vi "PLC.vi"(11 "Idx":i32) -> ()   [LabVIEW 2016]
doc: "Sound Analyzer queued state machine"
uses:
  PLC.Data.ctl
  PLC.Data.Status.ctl
  PLC.State.ctl
  PLC.Data.Sets.ctl
  LowLevel/PLC.DataBlock.PCstatus.ctl
  LowLevel/PLC.DataBlock.PCstatus.General.ctl
  LowLevel/PLC.DataBlock.PCstatus.Station.ctl
  LowLevel/PLC.DataBlock.PLCstatus.ctl
  LowLevel/PLC.DataBlock.PLCstatus.General.ctl
  LowLevel/PLC.DataBlock.PLCstatus.Station.ctl
  PLC.Action.ctl
  tools/CitTemplate/citTemplate.errData.ctl
  tools/EventLog/EventLog.EventSource.ctl
  Database/Database.Global.vi
  PLC.Global.vi
panel:
  out "action":T1=enum."-- PLC --"
  out "error.action":string
  out "error":errorcluster
  out "Data":T2={"Status"={"Idx"=0, "ConnRef"=0, "State"=enum."Off", "LiveBitTimer"=timestamp(0 s since 1904-01-01)}, "Sets"={"Enable"=FALSE, "IP"="", "Rack"=0, "Slot"=10000, "LifeBitTimer_s"=0.0, "DataBlockAddr_PCStatus"=0, "DataBlockAddr_PLCStatus"=1, "DataBlockAddr_PLCNewData"=[], "DataBlockSize_PLCNewData"=[], "DataBlockAddr_PLCChangeOver"=[], "DataBlockSize_PLCChangeOver"=[], "DataBlockAddr_PCChangeOver"=[], "DataBlockAddr_PLCCheckStatus"=[], "DataBlockSize_PLCCheckStatus"=[], "DataBlockAddr_PCCheckStatus"=[], "System"=""}, "PCstatus"={"General"={"LifeBit"=FALSE, "DbRun"=FALSE}, "Stations"=[]}, "PLCstatus"={"General"={"LifeBit"=FALSE}, "Stations"=[]}}
  out "_loop":i32(ring)=4
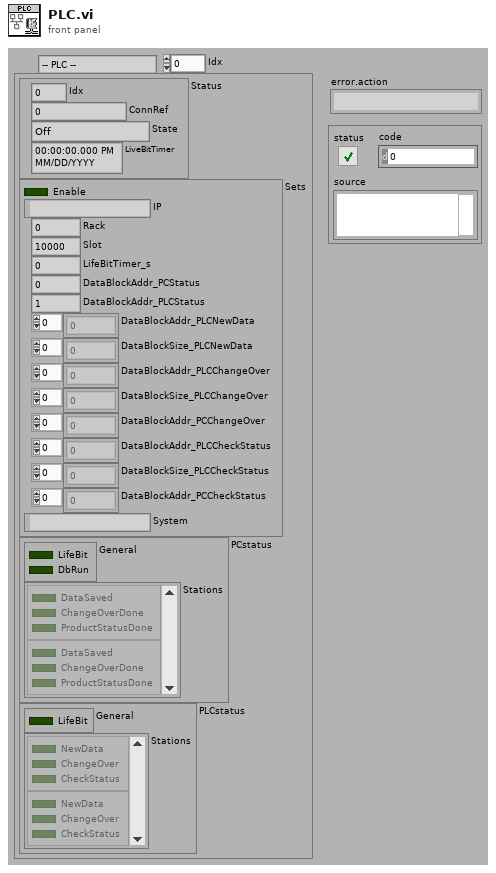
[diagram p1: front panel]
types:
  T1 = typedef "PLC.Action.ctl" = enum32{"idle", "constructor", "destructor", "-- PLC --", "Setup", "NewData", "ChangeOver", "CheckStatus"}
  T2 = typedef "PLC.Data.ctl" = cluster{"Status":T3, "Sets":T5, "PCstatus":T6, "PLCstatus":T9}
  T3 = typedef "PLC.Data.Status.ctl" = cluster{"Idx":i32, "ConnRef":u64, "State":T4, "LiveBitTimer":timestamp}
  T4 = typedef "PLC.State.ctl" = enum32{"Off", "Error", "Idle", "Run"}
  T5 = typedef "PLC.Data.Sets.ctl" = cluster{"Enable":bool, "IP":string, "Rack":i32, "Slot":i32, "LifeBitTimer_s":dbl, "DataBlockAddr_PCStatus":i32, "DataBlockAddr_PLCStatus":i32, "DataBlockAddr_PLCNewData":i32[], "DataBlockSize_PLCNewData":i32[], "DataBlockAddr_PLCChangeOver":i32[], "DataBlockSize_PLCChangeOver":i32[], "DataBlockAddr_PCChangeOver":i32[], "DataBlockAddr_PLCCheckStatus":i32[], "DataBlockSize_PLCCheckStatus":i32[], "DataBlockAddr_PCCheckStatus":i32[], "System":string}
  T6 = typedef "PLC.DataBlock.PCstatus.ctl" = cluster{"General":T7, "Stations":T8[]}
  T7 = typedef "PLC.DataBlock.PCstatus.General.ctl" = cluster{"LifeBit":bool, "DbRun":bool}
  T8 = typedef "PLC.DataBlock.PCstatus.Station.ctl" = cluster{"DataSaved":bool, "ChangeOverDone":bool, "ProductStatusDone":bool}
  T9 = typedef "PLC.DataBlock.PLCstatus.ctl" = cluster{"General":T10, "Stations":T11[]}
  T10 = typedef "PLC.DataBlock.PLCstatus.General.ctl" = cluster{"LifeBit":bool}
  T11 = typedef "PLC.DataBlock.PLCstatus.Station.ctl" = cluster{"NewData":bool, "ChangeOver":bool, "CheckStatus":bool}
  T12 = typedef "EventLog.EventSource.ctl" = enum16{"All", "Gui", "Ref", "File", "Arch", "Seq", "CPX", "DB", "Laser", "Scan.P", "Scan.O", "PLC"}
  T13 = typedef "citTemplate.errData.ctl" = cluster{"ts":timestamp, "src":T12, "instance":i32, "action":string, "error":errorcluster, "unconfirmed":bool}
  T14 = typedef "citTemplate.notifierHandle.ctl" = refnum<notifier>
  T15 = typedef "Database.Main.Data.Status.ctl" = cluster{"Run":bool, "Handle":i32, "ConnTS":timestamp, "DbTime":timestamp, "DbTimeCode":dbl, "DbTimeOffset":dbl}
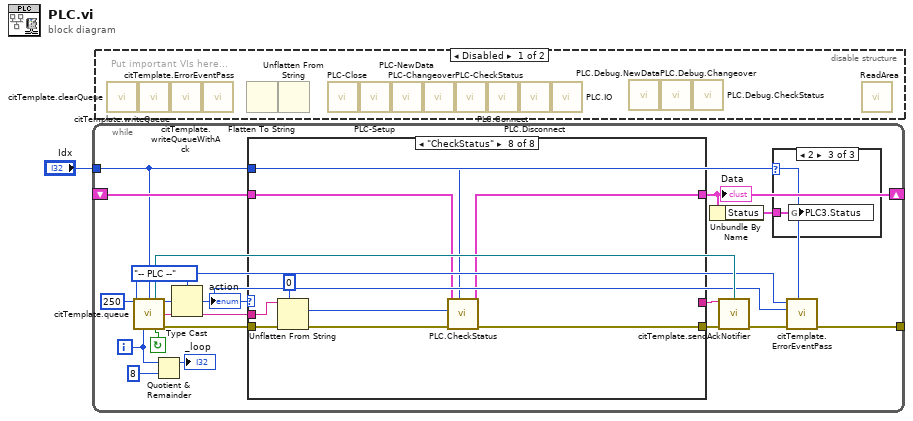
[diagram p0: block diagram]
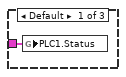
[diagram p2: hidden frame]
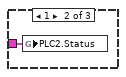
[diagram p3: hidden frame]
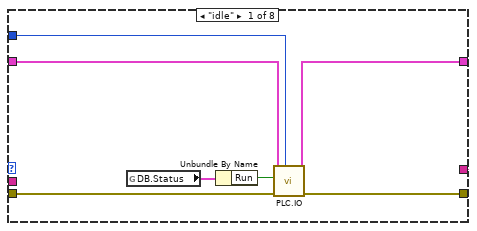
[diagram p4: hidden frame]
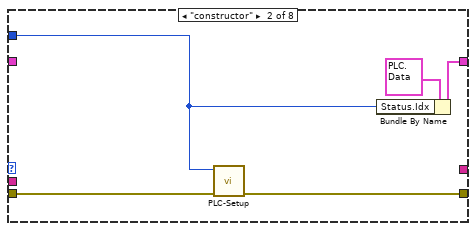
[diagram p5: hidden frame]
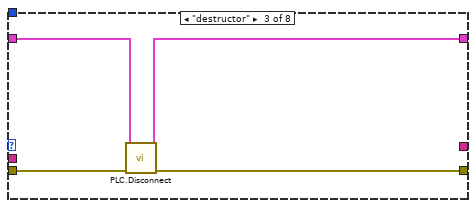
[diagram p6: hidden frame]
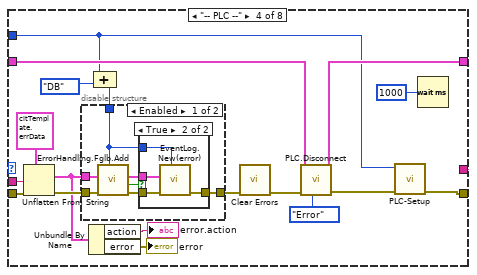
[diagram p7: hidden frame]
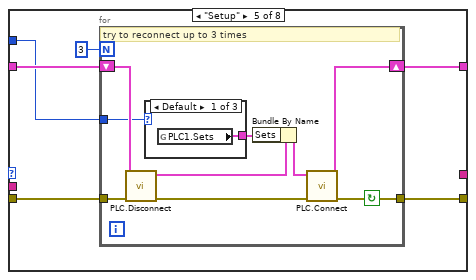
[diagram p10: hidden frame]
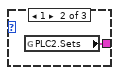
[diagram p11: hidden frame]
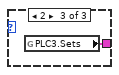
[diagram p12: hidden frame]
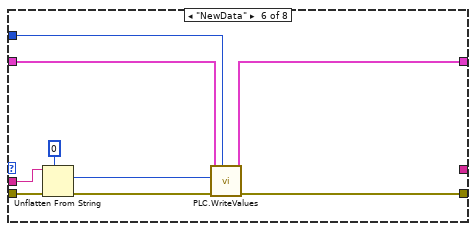
[diagram p13: hidden frame]
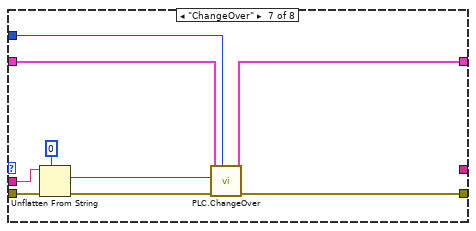
[diagram p14: hidden frame]
diagram:
  n1 = while {
    tunnel: [w9] -> _
    shift-right: [w6] -> _
    shift-left: _ -> [w7]
    tunnel: "Idx" -> [w2]
    i -> [w11]
    stop <- w16 continue-if-true
    w5 = PLC.Action."-- PLC --" ("Action")
    n2 = call "citTemplate.queue.vi"("ms timeout (250 ms)"=250, "instance (0)"=w2, "event enum"=w5, "iteration (-1)"=w11) -> ("notifierHandle out"=w15:T14, "event out"=w19:u32, "(flatten) data out"=w18:string, "continue"=w16:bool, "error out"=w17:errorcluster)  [unwired: 1 in, 6 out]
    n3 = Quotient & Remainder(x=w11, y=8) -> (x-y*floor(x/y)=→"_loop":i32)  [unwired: 1 out]
    n4 = Type Cast(type=w5, x=w19) -> (*(type *) &x=w10:T1)
    "action" <- w10
    n5 = case shown="\"CheckStatus\"" w10 {
      tunnel: w18 -> [_ _ _ w50 _ w91 w99 w108]
      tunnel: w17 -> [w28 w35 w39 w51 w76 w97 w101 w110]
      tunnel: ["" _ _ "" _ _ _ _] -> w14
      tunnel: [w27 w34 w38 w46 w75 w96 w106 w115] -> w4
      tunnel: [w26 w32 w36 w47 w74 w94 w104 w113] -> w6
      tunnel: w7 -> [w29 _ w37 w48 w73 w95 w105 w114]
      tunnel: w2 -> [w25 w31 _ w42 w71 w93 w103 w112]
      frame "idle" {
        n6 = global read "Database.Global.vi" "DB.Status"() -> (w24:T15)
        n7 = Unbundle By Name(w24) -> ("Run"=w23:bool)
        n8 = call "PLC.IO.vi"("Idx"=w25, "error in"=w28, "DbRun"=w23, "Data_in"=w29) -> ("error out"=w27:errorcluster, "Data_out"=w26:T2)  [unwired: 6 in]
      }
      frame "constructor" {
        n9 = call "PLC-Setup.vi"("error in"=w35, "Idx"=w31) -> ("error out"=w34:errorcluster)  [unwired: 9 in]
        n10 = Bundle By Name(cluster=T2 {"Status"={"Idx"=0, "ConnRef"=0, "State"=enum."Off", "LiveBitTimer"=timestamp(0 s since 1904-01-01)}, "Sets"={"Enable"=FALSE, "IP"="", "Rack"=0, "Slot"=10000, "LifeBitTimer_s"=0.0, "DataBlockAddr_PCStatus"=0, "DataBlockAddr_PLCStatus"=0, "DataBlockAddr_PLCNewData"=[], "DataBlockSize_PLCNewData"=[], "DataBlockAddr_PLCChangeOver"=[], "DataBlockSize_PLCChangeOver"=[], "DataBlockAddr_PCChangeOver"=[], "DataBlockAddr_PLCCheckStatus"=[], "DataBlockSize_PLCCheckStatus"=[], "DataBlockAddr_PCCheckStatus"=[], "System"=""}, "PCstatus"={"General"={"LifeBit"=FALSE, "DbRun"=FALSE}, "Stations"=[]}, "PLCstatus"={"General"={"LifeBit"=FALSE}, "Stations"=[]}} ("Data"), "Status.Idx"=w31) -> (w32:T2)
      }
      frame "destructor" {
        n11 = call "PLC.Disconnect.vi"("error in (no error)"=w39, "Data"=w37) -> ("error out"=w38:errorcluster, "Data out"=w36:T2)  [unwired: 8 in]
      }
      frame "-- PLC --" {
        n12 = Unflatten From String(type=T13 {"ts"=timestamp(0 s since 1904-01-01), "src"=enum."All", "instance"=0, "action"="", "error"={"status"=FALSE, "code"=0, "source"=""}, "unconfirmed"=FALSE} ("ErrData"), binary string=w50, error in (no error)=w51) -> (value=w54:T13, error out=w55:errorcluster)  [unwired: 2 in, 1 out]
        n13 = Unbundle By Name(w54) -> ("action"=→"error.action":string, "error"=→"error":errorcluster)
        n14 = Compound Arithmetic op=ADD(w42, EventLog.EventSource."DB" ("Event source")) -> (w41:i32)
        n15 = disable-structure shown="Enabled" {
          disable-tunnel: w55 -> [w64 w70]
          disable-tunnel: w54 -> [w63 _]
          disable-tunnel: [w62 w70] -> w49
          disable-tunnel: w41 -> [w59 _]
          frame Enabled {
            n16 = call "ErrorHandling.Fglb.Add.vi"("Event source"=w59, "error in (no error)"=w64, "Error in"=w63) -> ("error out"=w61:errorcluster, "changed?"=w60:bool)  [unwired: 7 in]
            n17 = case shown="True" w60 {
              tunnel: [w65 w69] -> w62
              tunnel: w63 -> [_ w68]
              tunnel: w61 -> [w65 w67]
              tunnel: w59 -> [_ w66]
              frame False {
              }
              frame True {
                n18 = call "EventLog.New(error).vi"("Source (All)"=w66, "error in"=w67, "ErrData"=w68) -> ("error out"=w69:errorcluster)  [unwired: 8 in]
              }
            }
          }
          frame Disabled {
          }
        }
        n19 = call <vilib>:"Clear Errors.vi"("error in (no error)"=w49) -> ("error out"=w43:errorcluster)  [unwired: 5 in, 1 out]
        n20 = call "PLC.Disconnect.vi"("State (Off)"=PLC.State."Error", "error in (no error)"=w43, "Data"=w48) -> ("error out"=w45:errorcluster, "Data out"=w47:T2)  [unwired: 7 in]
        n21 = call "PLC-Setup.vi"("error in"=w45, "Idx"=w42) -> ("error out"=w46:errorcluster)  [unwired: 9 in]
        n22 = Wait (ms)(milliseconds to wait=u32 1000) -> ()  [unwired: 1 out]
      }
      frame "Setup" {
        n23 = for {
          N: 3 -> [_]
          tunnel: w76 -> [w85]
          tunnel: [w78] -> w75
          shift-right: [w83] -> w74
          shift-left: w73 -> [w82]
          tunnel: w71 -> [w77]
          stop <- w78 continue-if-true
          # "try to reconnect up to 3 times"
          n24 = call "PLC.Disconnect.vi"("error in (no error)"=w85, "Data"=w82) -> ("error out"=w84:errorcluster, "Data out"=w80:T2)  [unwired: 8 in]
          n25 = case shown="Default" w77 {
            tunnel: [w86 w87 w88] -> w81
            frame Default {
              n26 = global read "PLC.Global.vi" "PLC1.Sets"() -> (w86:T5)
            }
            frame 1 {
              n27 = global read "PLC.Global.vi" "PLC2.Sets"() -> (w87:T5)
            }
            frame 2 {
              n28 = global read "PLC.Global.vi" "PLC3.Sets"() -> (w88:T5)
            }
          }
          n29 = Bundle By Name(cluster=w80, "Sets"=w81) -> (w79:T2)
          n30 = call "PLC.Connect.vi"("error in (no error)"=w84, "Data"=w79) -> ("error out"=w78:errorcluster, "Data out"=w83:T2)  [unwired: 8 in]
        }
      }
      frame "NewData" {
        n31 = Unflatten From String(type=0 ("Slot"), binary string=w91, error in (no error)=w97) -> (value=w89:i32, error out=w92:errorcluster)  [unwired: 2 in, 1 out]
        n32 = call "PLC.WriteValues.vi"("Idx"=w93, "error in"=w92, "Slot"=w89, "Data_in"=w95) -> ("error out"=w96:errorcluster, "Data_out"=w94:T2)  [unwired: 6 in]
      }
      frame "ChangeOver" {
        n33 = Unflatten From String(type=0 ("Slot"), binary string=w99, error in (no error)=w101) -> (value=w98:i32, error out=w100:errorcluster)  [unwired: 2 in, 1 out]
        n34 = call "PLC.ChangeOver.vi"("Idx"=w103, "error in"=w100, "Slot"=w98, "Data_in"=w105) -> ("error out"=w106:errorcluster, "Data_out"=w104:T2)  [unwired: 6 in]
      }
      frame "CheckStatus" {
        n35 = Unflatten From String(type=0 ("Slot"), binary string=w108, error in (no error)=w110) -> (value=w107:i32, error out=w109:errorcluster)  [unwired: 2 in, 1 out]
        n36 = call "PLC.CheckStatus.vi"("Idx"=w112, "error in"=w109, "Slot"=w107, "Data_in"=w114) -> ("error out"=w115:errorcluster, "Data_out"=w113:T2)  [unwired: 6 in]
      }
    }
    "Data" <- w6
    n37 = Unbundle By Name(w6) -> ("Status"=w3:T3)
    n38 = call "citTemplate.sendAckNotifier.vi"("notification data"=w14, "notifierHandle in"=w15, "error in"=w4) -> ()  [unwired: 13 out]
    n39 = case shown="2" w2 {
      tunnel: w3 -> [w20 w21 w22]
      frame Default {
        n40 = global write "PLC.Global.vi" "PLC1.Status"(w20) -> ()
      }
      frame 1 {
        n41 = global write "PLC.Global.vi" "PLC2.Status"(w21) -> ()
      }
      frame 2 {
        n42 = global write "PLC.Global.vi" "PLC3.Status"(w22) -> ()
      }
    }
    n43 = call "citTemplate.ErrorEventPass.vi"("instance"=w2, "error in"=w4, "action of error"=w10, "event in"=w5) -> ("error out"=w9:errorcluster)  [unwired: 1 in, 6 out]
  }
  n44 = disable-structure shown="Disabled" {
    frame Disabled {
      # "Put important VIs here..."
      n45 = call "citTemplate.clearQueue.vi"() -> ()  [unwired: 14 in, 2 out]
      n46 = call "citTemplate.writeQueue.vi"() -> ()  [unwired: 15 in, 1 out]
      n47 = call "citTemplate.writeQueueWithAck.vi"() -> ()  [unwired: 13 in, 3 out]
      n48 = call "citTemplate.ErrorEventPass.vi"() -> ()  [unwired: 11 in, 1 out]
      n49 = Flatten To String() -> ()  [unwired: 4 in, 3 out]
      n50 = Unflatten From String() -> ()  [unwired: 5 in, 3 out]
      n51 = call "PLC-Close.vi"() -> ()  [unwired: 11 in, 1 out]
      n52 = call "PLC-Setup.vi"() -> ()  [unwired: 11 in, 1 out]
      n53 = call "PLC-NewData.vi"() -> ()  [unwired: 11 in, 1 out]
      n54 = call "PLC-Changeover.vi"() -> ()  [unwired: 11 in, 1 out]
      n55 = call "PLC-CheckStatus.vi"() -> ()  [unwired: 11 in, 1 out]
      n56 = call "PLC.Connect.vi"() -> ()  [unwired: 10 in, 2 out]
      n57 = call "PLC.Disconnect.vi"() -> ()  [unwired: 10 in, 2 out]
      n58 = call "PLC.IO.vi"() -> ()  [unwired: 10 in, 2 out]
      n59 = call "PLC.Debug.NewData.vi"() -> ()  [unwired: 10 in, 2 out]
      n60 = call "PLC.Debug.Changeover.vi"() -> ()  [unwired: 10 in, 2 out]
      n61 = call "PLC.Debug.CheckStatus.vi"() -> ()  [unwired: 10 in, 2 out]
      n62 = call "ReadArea.vi"() -> ()  [unwired: 12 in]
    }
    frame Enabled {
    }
  }
